vi "UI Configure Panel.vi"(8 "error in (no error)":errorcluster, 11 "Button_UI in":refnum<class "Button_UI.lvclass">) -> (0 "error out":errorcluster, 3 "Button_UI out":refnum<class "Button_UI.lvclass">)   [LabVIEW 2015, in "Button_UI.lvclass"]
uses:
  Button_UI.lvclass
  GUI Control/Type Definition/UI Configuration State Variable.ctl
  Button_UI.lvclass/Button_UI.ctl
  <vilib>/Utility/error.llb/Error Cluster From Error Code.vi
  <vilib>/ErrorRing/Error Ring.xnode
panel:
  in  "OK Button":bool
  in  "UI Style":string(combo)
  in  "Protocol":string
  in  "UI_Name":string
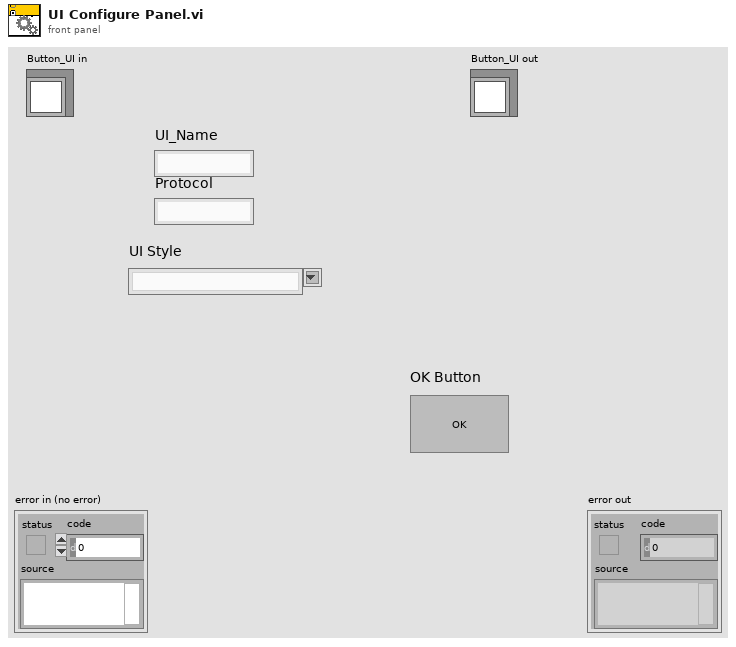
[diagram p1: front panel]
types:
  T1 = typedef "UI Configuration State Variable.ctl" = enum16{"Initialize", "Panel On", "Working", "Panel Off", "End"}
  T2 = enum32{"Invalid", "Standard", "Closed", "Hidden", "Minimized", "Maximized"}
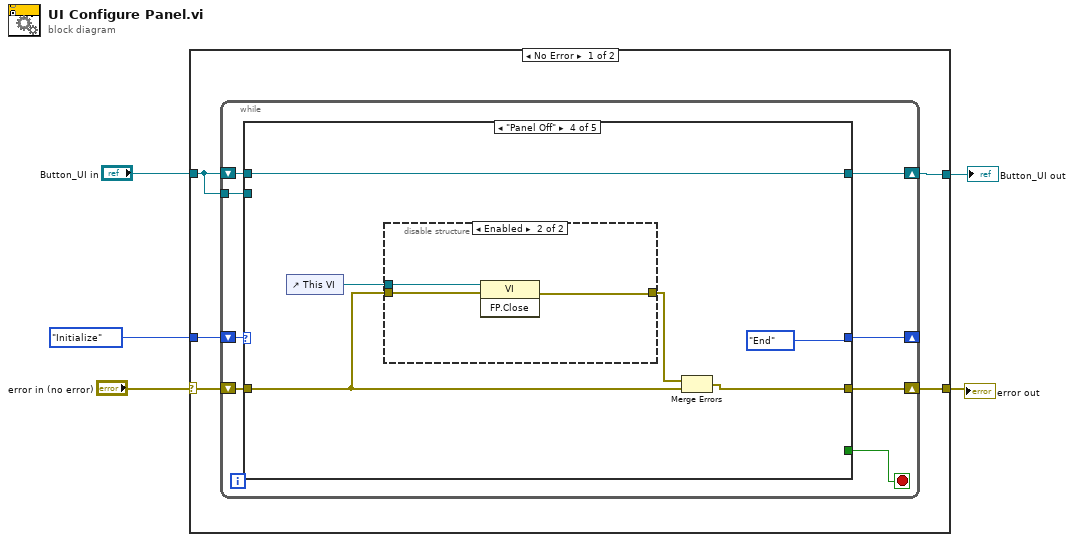
[diagram p0: block diagram]
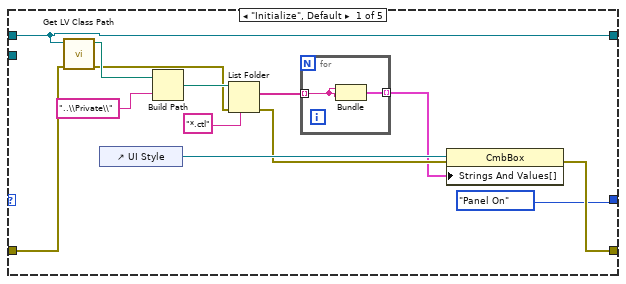
[diagram p2: hidden frame]
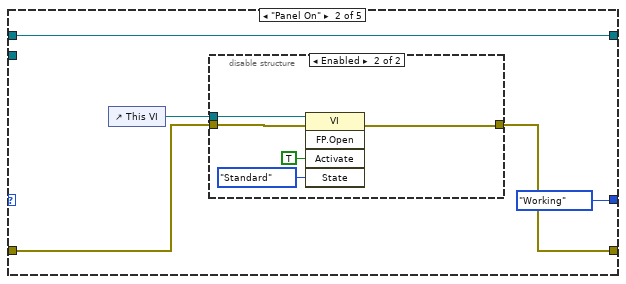
[diagram p3: hidden frame]
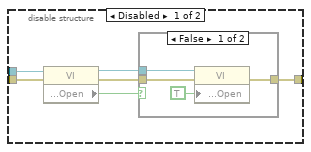
[diagram p4: hidden frame]
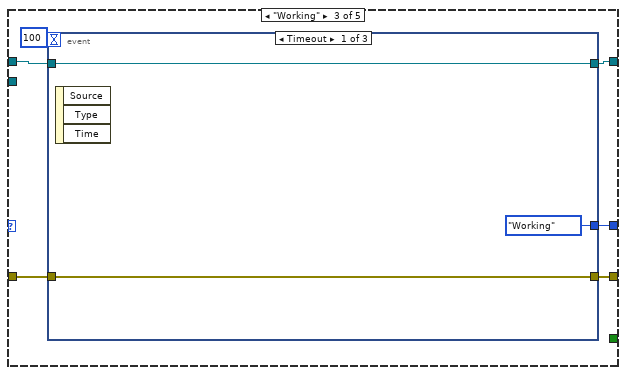
[diagram p6: hidden frame]
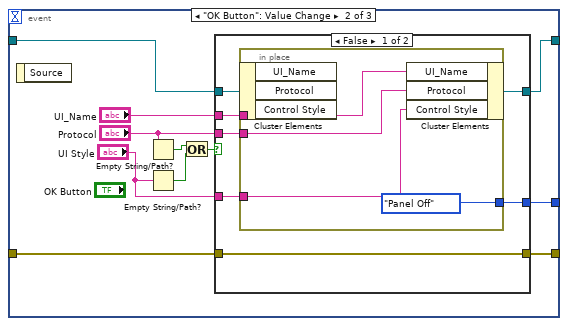
[diagram p7: hidden frame]
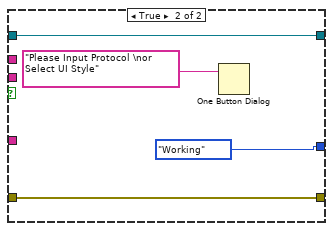
[diagram p8: hidden frame]
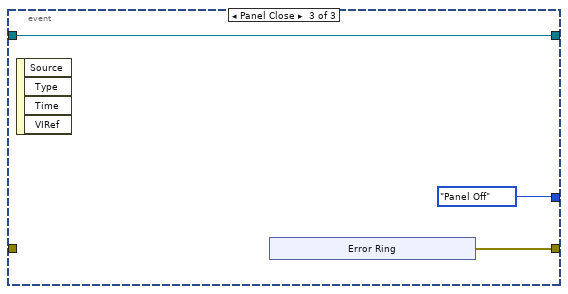
[diagram p9: hidden frame]
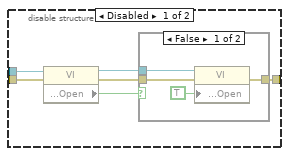
[diagram p10: hidden frame]
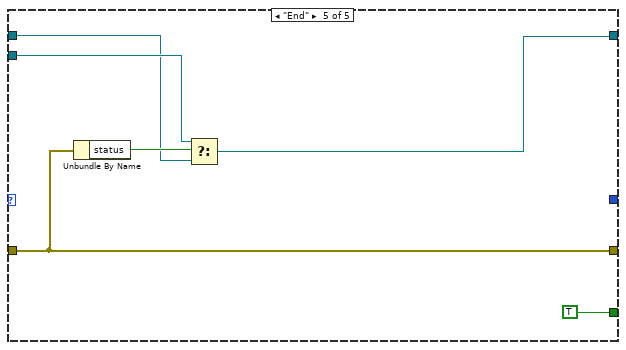
[diagram p12: hidden frame]
diagram:
  n1 = case shown="No Error" "error in (no error)" {
    selector: "error in (no error)" -> [w9 w125]
    tunnel: UI_Configuration_State_Variable."Initialize" -> [w10 _]
    tunnel: "Button_UI in" -> [w6 w124]
    tunnel: [w8 w124] -> w2
    tunnel: [w7 w125] -> w1
    frame No Error {
      n2 = while {
        shift-right: [w15] -> w7
        shift-left: w9 -> [w16]
        shift-right: [w14] -> _
        shift-left: w10 -> [w17]
        shift-right: [w13] -> w8
        shift-left: w6 -> [w18]
        tunnel: w6 -> [w11]
        stop <- w12 stop-if-true
        n3 = case shown="\"Panel Off\"" w17 {
          tunnel: w18 -> [w19 w38 w60 w103 w119]
          tunnel: w16 -> [w26 w36 w59 w99 w122]
          tunnel: [w23 w35 w56 w102 w122] -> w15
          tunnel: [UI_Configuration_State_Variable."Panel On" UI_Configuration_State_Variable."Working" w58 UI_Configuration_State_Variable."End" _] -> w14
          tunnel: [w19 w38 w57 w103 w118] -> w13
          tunnel: [_ _ _ _ TRUE] -> w12
          tunnel: w11 -> [_ _ _ _ w120]
          frame "Initialize", Default {
            n4 = call <vilib>:"Get LV Class Path.vi"("error in (no error)"=w26, "object"=w19) -> ("error out"=w27:errorcluster, "class path"=w31:path)  [unwired: 8 in]
            n5 = control-ref of="UI Style"() -> (w25:refnum<vi>)
            n6 = Build Path(base path=w31, name or relative path="..\\Private\\") -> (appended path=w29:path)
            n7 = List Folder(path=w29, pattern="*.ctl", error in=w27) -> (filenames=w22:string[], error out=w24:errorcluster)  [unwired: 1 in, 2 out]
            n8 = for {
              tunnel: w22 -> [w33] mode=indexing
              tunnel: [w32] -> w21 mode=indexing
              n9 = Bundle(w33, w33) -> (w32:cluster{string, string})  [unwired: 1 in]
            }
            n10 = property class="CmbBox"(reference=w25, error in=w24, "Strings And Values[]"=w21) -> (error out=w23:errorcluster)  [unwired: 1 out]
          }
          frame "Panel On" {
            n11 = control-ref of="This VI"() -> (w37:refnum<vi>)
            n12 = disable-structure shown="Enabled" {
              disable-tunnel: w37 -> [w44 w54]
              disable-tunnel: w36 -> [w43 w53]
              disable-tunnel: [w39 w50] -> w35
              frame Disabled {
                n13 = property class="VI"(reference=w44, error in=w43) -> (reference out=w40:refnum<vi>, error out=w41:errorcluster, "Front Panel.Open"=w42:bool)
                n14 = case shown="False" w42 {
                  tunnel: w41 -> [w47 w49]
                  tunnel: w40 -> [w48 _]
                  tunnel: [w45 w49] -> w39
                  frame False {
                    n15 = property class="VI"(reference=w48, error in=w47, "Front Panel.Open"=TRUE ("Front Panel Window:Open")) -> (error out=w45:errorcluster)  [unwired: 1 out]
                  }
                  frame True {
                  }
                }
              }
              frame Enabled {
                n16 = invoke class="VI" method="FP.Open"(reference=w54, error in=w53, "Activate"=TRUE ("Activate?"), "State"=T2."Standard") -> (error out=w50:errorcluster)  [unwired: 1 in, 4 out]
              }
            }
          }
          frame "Working" {
            n17 = event shown="[0] Timeout" {
              selector: _ -> [_ _ _]
              dyn-events: _ -> [_ _ _]
              timeout: 100 -> [_ _ _]
              tunnel: w60 -> [w63 w66 w92]
              tunnel: w59 -> [w62 w71 _]
              tunnel: [UI_Configuration_State_Variable."Working" w70 UI_Configuration_State_Variable."Panel Off"] -> w58
              tunnel: [w63 w65 w92] -> w57
              tunnel: [w62 w64 w91] -> w56
              event Timeout {
                n18 = event-data() -> ()  [unwired: 1 in, 3 out]
              }
              event "OK Button": Value Change {
                n19 = event-data() -> ()  [unwired: 1 in, 1 out]
                n20 = Empty String/Path?(string/path="Protocol") -> (empty?=w74:bool)
                n21 = Empty String/Path?(string/path="UI Style") -> (empty?=w73:bool)
                n22 = Or(x=w74, y=w73) -> (x .or. y?=w72:bool)
                n23 = case shown="False" w72 {
                  tunnel: w71 -> [w75 w86]
                  tunnel: [w76 UI_Configuration_State_Variable."Working"] -> w70
                  tunnel: "UI_Name" -> [w80 _]
                  tunnel: "Protocol" -> [w79 _]
                  tunnel: "UI Style" -> [w78 _]
                  tunnel: w66 -> [w81 w88]
                  tunnel: [w77 w88] -> w65
                  tunnel: [w75 w86] -> w64
                  frame False {
                    n24 = in-place {
                      in-place-border: w80 -> [w85]
                      in-place-border: w79 -> [w84]
                      in-place-border: w78 -> [w83]
                      in-place-border: [UI_Configuration_State_Variable."Panel Off"] -> w76
                      n25 = in-place-cluster #1(w81) -> ()  [unwired: 3 out]
                      n26 = in-place-cluster #1("UI_Name"=w85, "Protocol"=w84, "Control Style"=w83) -> (w77:refnum<class "Button_UI.lvclass">)
                    }
                  }
                  frame True {
                    n27 = One Button Dialog(message="Please Input Protocol \nor Select UI Style") -> ()  [unwired: 1 in, 1 out]
                  }
                }
              }
              event Panel Close {
                n28 = event-data() -> ()  [unwired: 1 in, 4 out]
                n29 = xnode "Error Ring"() -> ("error out"=w91:errorcluster)
              }
            }
          }
          frame "Panel Off" {
            n30 = control-ref of="This VI"() -> (w100:refnum<vi>)
            n31 = disable-structure shown="Enabled" {
              disable-tunnel: w100 -> [w109 w116]
              disable-tunnel: w99 -> [w108 w115]
              disable-tunnel: [w104 w117] -> w98
              frame Disabled {
                n32 = property class="VI"(reference=w109, error in=w108) -> (reference out=w105:refnum<vi>, error out=w106:errorcluster, "Front Panel.Open"=w107:bool)
                n33 = case shown="False" w107 {
                  tunnel: w106 -> [w112 w114]
                  tunnel: w105 -> [w113 _]
                  tunnel: [w110 w114] -> w104
                  frame False {
                    n34 = property class="VI"(reference=w113, error in=w112, "Front Panel.Open"=TRUE ("Front Panel Window:Open")) -> (error out=w110:errorcluster)  [unwired: 1 out]
                  }
                  frame True {
                  }
                }
              }
              frame Enabled {
                n35 = invoke class="VI" method="FP.Close"(reference=w116, error in=w115) -> (error out=w117:errorcluster)  [unwired: 1 in, 2 out]
              }
            }
            n36 = Merge Errors(w98, w99) -> (w102:errorcluster)
          }
          frame "End" {
            n37 = Unbundle By Name(w122) -> ("status"=w121:bool)
            n38 = Select(t=w120, s=w121, f=w119) -> (s? t:f=w118:refnum<class "Button_UI.lvclass">)
          }
        }
      }
    }
    frame Error {
    }
  }
  "error out" <- w1
  "Button_UI out" <- w2
